vi "IniToken LoadInfoFromFile.vi"(8 "error in (no error)":errorcluster, 11 "Path":path=path "D:/Dropbox/_workingOn/LabVIEW-Developing-QuickDrops/src/user.lib/_NEVSTOP/_LabVIEW.ini/test.iniToken") -> (0 "error out":errorcluster, 3 "Array":T2(array[cluster]))   [LabVIEW 2015]
uses:
  Def-IniTokenCluster.ctl
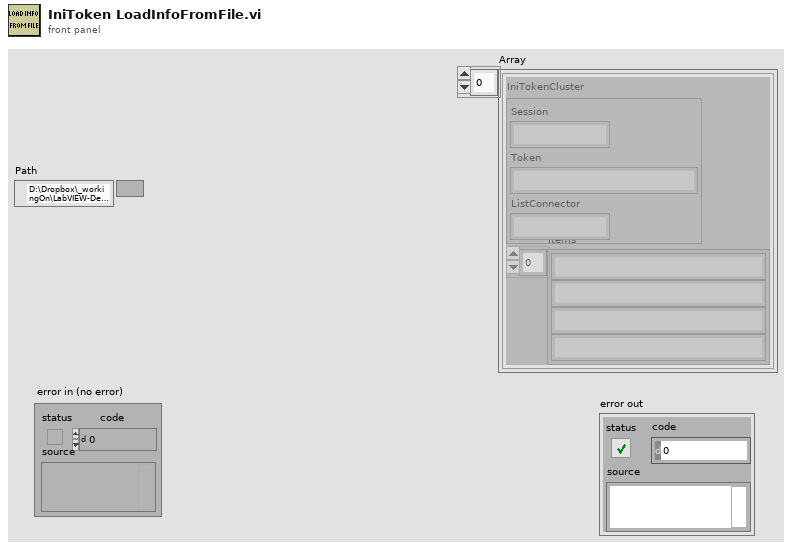
[diagram p1: front panel]
types:
  T1 = typedef "Def-IniTokenCluster.ctl" = cluster{"Session":string, "Token":string, "ListConnector":string}
  T2 = cluster{"IniTokenCluster":T1, "Items":string[]}[]
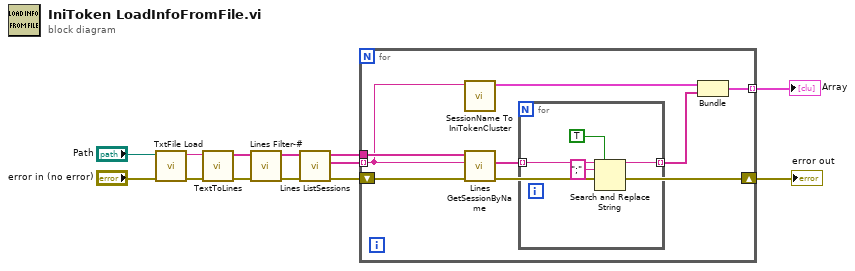
[diagram p0: block diagram]
diagram:
  n1 = call "TxtFile Load.vi"("error in (no error)"="error in (no error)", "Path"="Path") -> ("error out"=w8:errorcluster, "text"=w12:string)  [unwired: 8 in]
  n2 = call "TextToLines.vi"("error in (no error)"=w8, "string"=w12) -> ("error out"=w7:errorcluster, "Lines"=w11:string[])  [unwired: 8 in]
  n3 = call "Lines Filter-#.vi"("error in (no error)"=w7, "Lines"=w11) -> ("error out"=w6:errorcluster, "Config Text List"=w10:string[])  [unwired: 8 in]
  n4 = call "Lines ListSessions.vi"("error in (no error)"=w6, "Config Text List"=w10) -> ("error out"=w5:errorcluster, "Sessions"=w4:string[], "Config Text List out"=w9:string[])  [unwired: 7 in]
  n5 = for {
    tunnel: w9 -> [w21]
    tunnel: w4 -> [w19] mode=indexing
    tunnel: [w17] -> w3 mode=indexing
    shift-right: [w16] -> w2
    shift-left: w5 -> [w20]
    n6 = call "SessionName To IniTokenCluster.vi"("trimmed string"=w19) -> ("IniTokenCluster"=w18:T1)  [unwired: 10 in]
    n7 = call "Lines GetSessionByName.vi"("error in (no error)"=w20, "[] Session Name"=w19, "Config Text List"=w21) -> ("error out"=w16:errorcluster, "Session"=w15:string[])  [unwired: 6 in, 1 out]
    n8 = for {
      tunnel: w15 -> [w25] mode=indexing
      tunnel: [w24] -> w14 mode=indexing
      n9 = Search and Replace String(replace all?=TRUE ("replace all? (F)"), input string=w25, search string=";") -> (result string=w24:string)  [unwired: 5 in, 3 out]
    }
    n10 = Bundle("IniTokenCluster"=w18, w14) -> (w17:cluster{"IniTokenCluster":T1, string[]})  [unwired: 1 in]
  }
  "Array" <- w3
  "error out" <- w2
